vi "Dye Recipe Table Step by Index.vi"(8 "error in (no error)":errorcluster, 9 "Dye Color":u32(colorbox), 10 "Index":u64, 11 "Kitchen Actor in":refnum<class "Kitchen Actor.lvclass">) -> (0 "error out":errorcluster, 3 "Kitchen Actor out":refnum<class "Kitchen Actor.lvclass">)   [LabVIEW 2024, in "Kitchen Actor.lvlib" / "Kitchen Actor.lvclass"]
uses:
  Kitchen Actor.lvclass
  Kitchen Actor.lvclass/Kitchen Actor.ctl
  <vilib>/Utility/miscctls.llb/LVRowAndColumnTypeDef.ctl
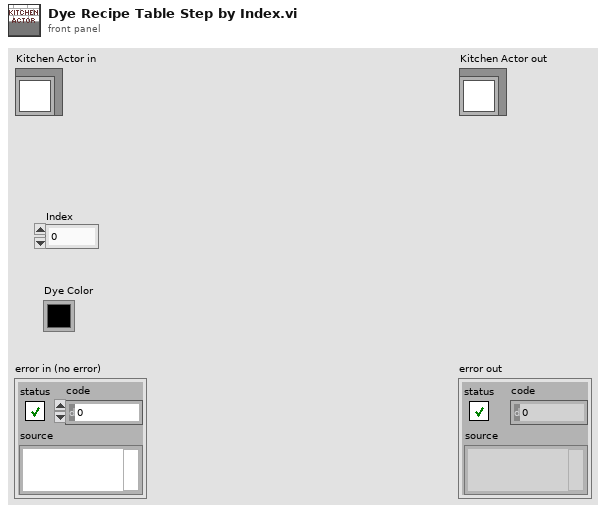
[diagram p1: front panel]
types:
  T1 = typedef "LVRowAndColumnTypeDef.ctl" = cluster{"Row":i32, "Column":i32}
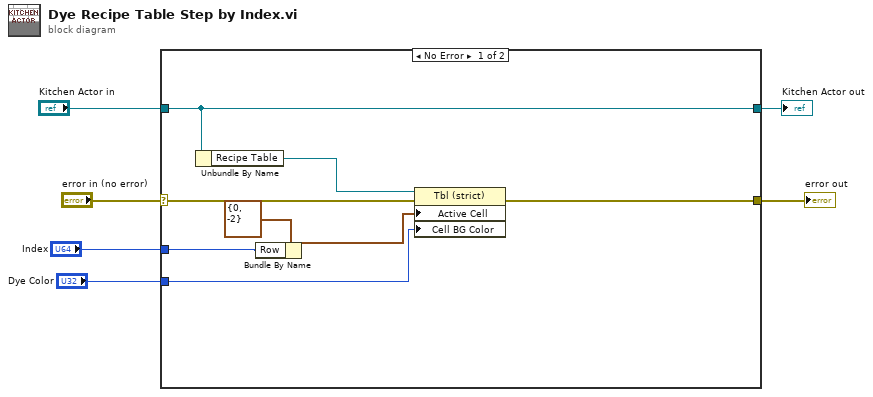
[diagram p0: block diagram]
diagram:
  n1 = case shown="No Error" "error in (no error)" {
    selector: "error in (no error)" -> [w14 w16]
    tunnel: [w12 w16] -> w5
    tunnel: [w13 w15] -> w3
    tunnel: "Kitchen Actor in" -> [w13 w15]
    tunnel: "Dye Color" -> [w10 _]
    tunnel: "Index" -> [w7 _]
    frame No Error {
      n2 = Unbundle By Name(w13) -> ("Recipe Table"=w11:refnum<vi>)
      n3 = Bundle By Name(cluster=T1 {"Row"=0, "Column"=-2} ("Active Cell:Active Cell"), "Row"=w7) -> (w9:T1)
      n4 = property class="Tbl (strict)"(reference=w11, error in=w14, "Active Cell"=w9, "Cell BG Color"=w10) -> (error out=w12:errorcluster)  [unwired: 1 out]
    }
    frame Error {
    }
  }
  "error out" <- w5
  "Kitchen Actor out" <- w3
